vi "synnax_client_smoke_test.vi"() -> ()   [LabVIEW 2026]
uses:
  lvlib/synnax_clib.lvlib
panel:
  in  "Value":dbl
  in  "password":string="seldon"
  in  "username":string="synnax"
  in  "port":u16=9090
  in  "host":string="localhost"
  out "error out":errorcluster
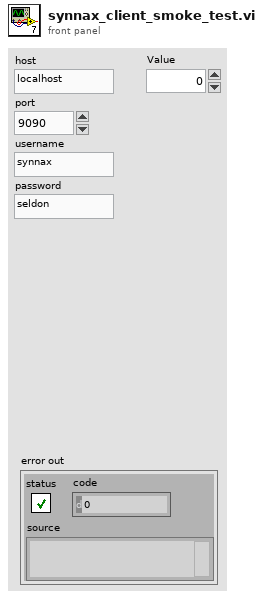
[diagram p1: front panel]
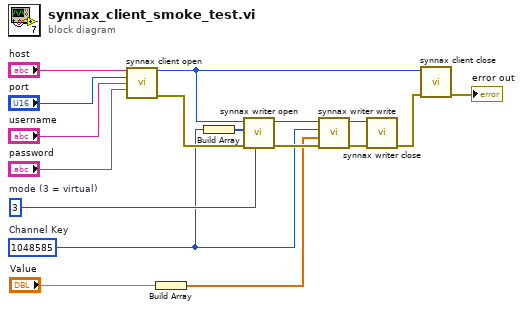
[diagram p0: block diagram]
diagram:
  w8 = 3  # mode (3 = virtual)
  w7 = u32 1048585  # Channel Key
  n1 = call "synnax client open.vi"("host"="host", "port"="port", "username"="username", "password"="password") -> ("client out"=w10:u64, "error out"=w13:errorcluster)  [unwired: 10 in]
  n2 = Build Array("Value") -> (w5:dbl[])
  n3 = Build Array(w7) -> (w9:u32[])
  n4 = call "synnax writer open.vi"("mode (Default)"=w8, "error in (no error)"=w13, "channels"=w9, "client in"=w10) -> ("error out"=w12:errorcluster, "writer out"=w3:u64)  [unwired: 6 in]
  n5 = call "synnax writer write.vi"("error in (no error)"=w12, "data"=w5, "channel"=w7, "writer"=w3) -> ("error out"=w1:errorcluster, "writer out"=w2:u64)  [unwired: 6 in]
  n6 = call "synnax writer close.vi"("error in (no error)"=w1, "writer"=w2) -> ("error out"=w11:errorcluster)  [unwired: 9 in]
  n7 = call "synnax client close.vi"("error in (no error)"=w11, "client"=w10) -> ("error out"=→"error out":errorcluster)  [unwired: 9 in]
